vi "daqio_Fire_Event.vi"(7 "Event Key":string, 8 "error in (no error)":errorcluster, 9 "Event Value":string, 10 "Event Date and Time":timestamp, 11 "daq.io type in":T1={"daq.io ref"=refnum, "daq.io API Base"="http://dashboard.daq.io/api/v1", "Device Type Key"="", "Device Key"="", "Account ID"="", "online"=FALSE}) -> (0 "error out":errorcluster, 3 "daq.io type out":T1={"daq.io ref"=refnum, "daq.io API Base"="http://dashboard.daq.io/api/v1", "Device Type Key"="", "Device Key"="", "Account ID"="", "online"=FALSE})   [LabVIEW 2013, in "daqio minimal.lvlib"]
doc: "This VI will Fire an Event for the given Event Key. If the Event Key does not exist, it will create a new Event on the device. Every event fired will have a timestamp and a value associated with it. Events can be of any type and will be reflected on the \"Events\" page on daq.io. to retrieve all events that occured, use \"Get Device Events\"."
uses:
  daqio minimal.lvlib
  <vilib>/Easy HTTP Client/HTTP Header.ctl
  _typedefs/daqio-Type.ctl
  <vilib>/httpClient/ClientHandle.ctl
  _typedefs/daqio-Event-Def-Min.ctl
  _typedefs/FGV_commands.ctl
  _typedefs/daqio-Buffer-Commands.ctl
  <vilib>/Easy HTTP Client/Easy HTTP.lvlib
  <vilib>/httpClient/LabVIEWHTTPClient.lvlib
panel:
  out "JSON string":string
  out "headers":T3[](array[typedef])
  out "body":string
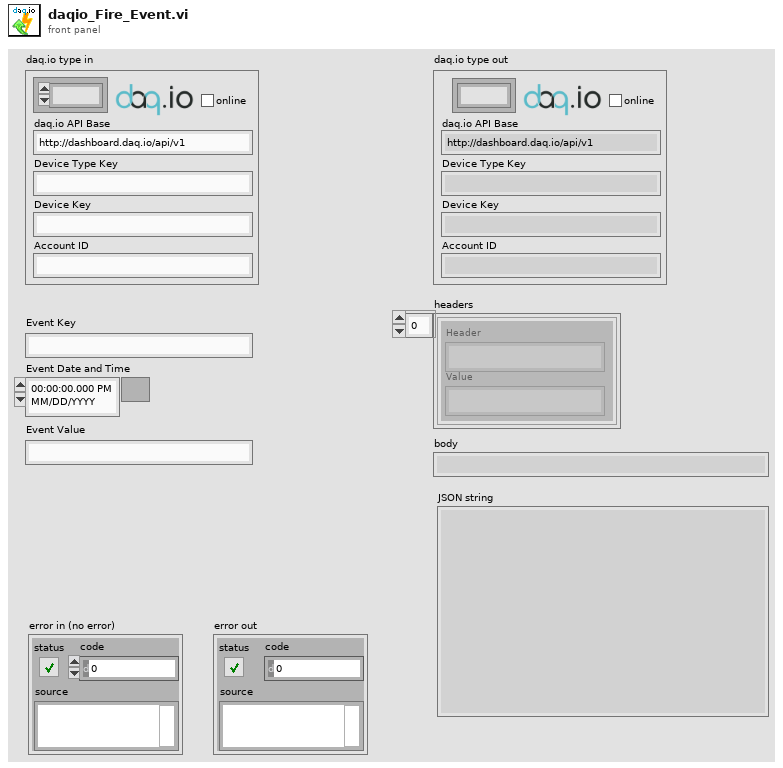
[diagram p1: front panel]
types:
  T1 = typedef "daqio minimal.lvlib/daqio-Type.ctl" = cluster{"daq.io ref":T2, "daq.io API Base":string, "Device Type Key":string, "Device Key":string, "Account ID":string, "online":bool}
  T2 = typedef "LabVIEWHTTPClient.lvlib/ClientHandle.ctl" = refnum<k1>
  T3 = typedef "Easy HTTP.lvlib/HTTP Header.ctl" = cluster{"Header":string, "Value":string}
  T4 = typedef "daqio minimal.lvlib/FGV_commands.ctl" = enum16{"Init / update", "Edit Item", "Find or Add Item", "Remove Item", "Delete All"}
  T5 = typedef "daqio minimal.lvlib/daqio-Event-Def-Min.ctl" = cluster{"event_type":string, "time":string, "value":string}
  T6 = typedef "daqio minimal.lvlib/daqio-Buffer-Commands.ctl" = enum16{"Add to Buffer", "Post from Buffer", "Clear Buffer", "Init"}
  T7 = typedef "daqio minimal.lvlib/daqio-Device-Type-Info-return.ctl" = cluster{"channel_types":T8[], "devices":T9[], "label":string, "event_types":T10[], "key":string, "tag_types":T11[], "id":string, "permissions":cluster{"write":string[], "read":string[]}}
  T8 = typedef "daqio minimal.lvlib/daqio-Channel-Type-POST-return.ctl" = cluster{"device_type_id":string, "id":string, "key":string, "label":string, "data_type":string, "permissions":cluster{"write":string[], "read":string[]}}
  T9 = typedef "daqio minimal.lvlib/daqio-Device.ctl" = cluster{"permissions":cluster{"write":string[], "read":string[]}, "id":string, "label":string, "key":string, "device_type_id":string, "tags":cluster{"key":string, "value":string}[], "files":string[]}
  T10 = typedef "daqio minimal.lvlib/daqio-Event-Type.ctl" = cluster{"device_type_id":string, "permissions":cluster{"read":string[], "write":string[]}, "id":string, "key":string, "label":string}
  T11 = typedef "daqio minimal.lvlib/daqio-Tag-Type-POST-return.ctl" = cluster{"label":string, "id":string, "device_type_id":string, "permissions":cluster{"write":string[], "read":string[]}, "default":string, "key":string}
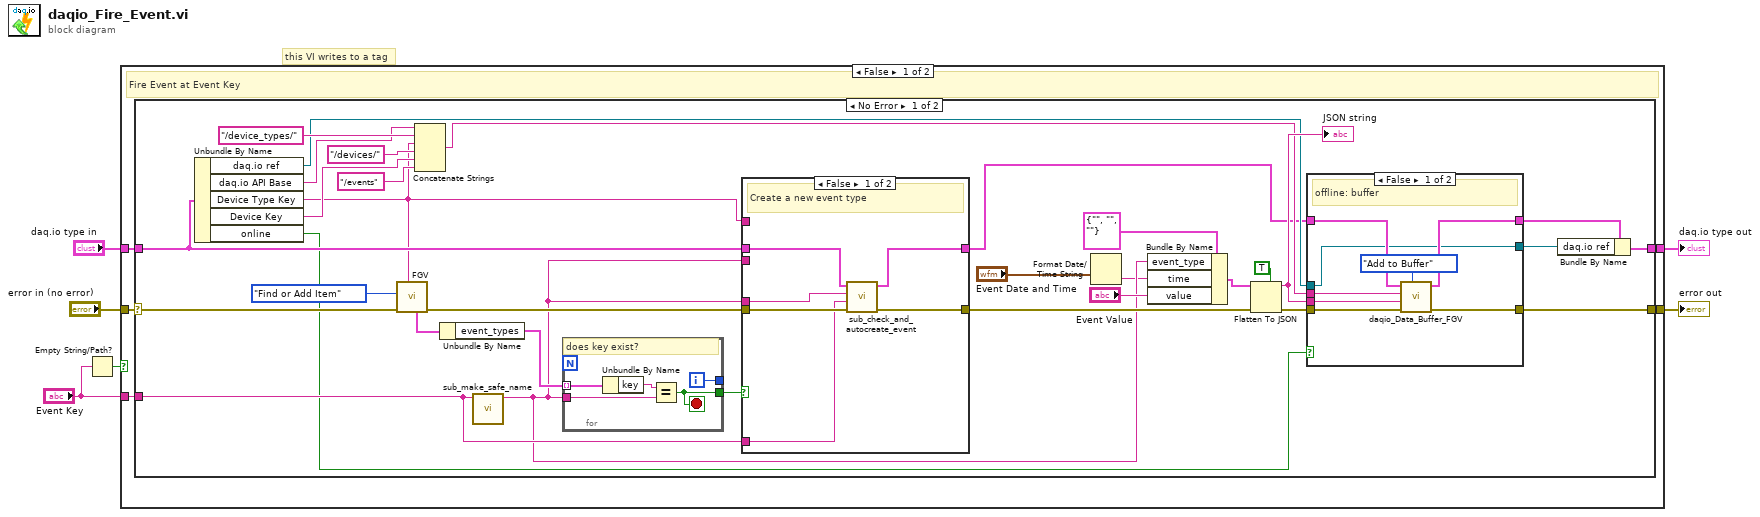
[diagram p0: block diagram]
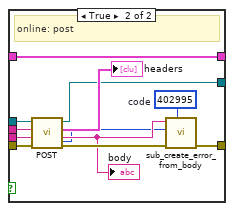
[diagram p2: hidden frame]
diagram:
  # "this VI writes to a tag"
  n1 = Empty String/Path?(string/path="Event Key") -> (empty?=w2:bool)
  n2 = case shown="False" w2 {
    tunnel: [w11 w80] -> w6
    tunnel: [w10 w79] -> w5
    tunnel: "error in (no error)" -> [w9 w79]
    tunnel: "daq.io type in" -> [w8 w80]
    tunnel: "Event Key" -> [w7 _]
    frame False {
      # "Fire Event at Event Key"
      n3 = case shown="No Error" w9 {
        selector: w9 -> [w27 w77]
        tunnel: [w35 w78] -> w11
        tunnel: [w33 w77] -> w10
        tunnel: w8 -> [w26 w78]
        tunnel: w7 -> [w18 _]
        frame No Error {
          n4 = Unbundle By Name(w26) -> ("daq.io ref"=w37:T2, "daq.io API Base"=w34:string, "Device Type Key"=w24:string, "Device Key"=w32:string, "online"=w16:bool)
          n5 = call "FGV.vi"("Dev Type Key"=w24, "error in (no error)"=w27, "Action"=FGV_commands."Find or Add Item") -> ("error out"=w28:errorcluster, "Dev Type out"=w29:T7)  [unwired: 4 in, 3 out]
          n6 = Concatenate Strings(w34, "/device_types/", w24, "/devices/", w32, "/events") -> (w41:string)
          n7 = Unbundle By Name(w29) -> ("event_types"=w23:T10[])
          n8 = call "sub_make_safe_name.vi"("Input String"=w18) -> ("Safe Output String"=w17:string)  [unwired: 10 in]
          n9 = for {
            tunnel: w23 -> [w76] mode=indexing
            tunnel: w17 -> [w74]
            tunnel: [w73] -> w25
            tunnel: [w72] -> _
            i -> [w72]
            stop <- w73 stop-if-true
            # "does key exist?"
            n10 = Unbundle By Name(w76) -> ("key"=w75:string)
            n11 = Equal?(x=w75, y=w74) -> (x = y?=w73:bool)
          }
          n12 = case shown="False" w25 {
            tunnel: w17 -> [w66 _]
            tunnel: w28 -> [w69 w71]
            tunnel: w26 -> [w68 w70]
            tunnel: [w67 w70] -> w15
            tunnel: [w64 w71] -> w20
            tunnel: w24 -> [_ _]
            tunnel: w17 -> [_ _]
            tunnel: w18 -> [w65 _]
            frame False {
              # "Create a new event type"
              n13 = call "sub_check_and_autocreate_event.vi"("error in (no error)"=w69, "new Event Label"=w65, "Event Key to Create or Update"=w66, "daq.io type in in"=w68) -> ("error out"=w64:errorcluster, "daq.io type out"=w67:T1)  [unwired: 5 in, 1 out]
            }
            frame True {
              # "Key was found in the existing device types"
            }
          }
          n14 = Format Date/Time String(seconds (now)="Event Date and Time") -> (date/time string=w13:string)  [unwired: 2 in]
          n15 = Bundle By Name(cluster=T5 {"event_type"="", "time"="", "value"=""} ("Devices"), "event_type"=w17, "time"=w13, "value"="Event Value") -> (w21:T5)
          n16 = Flatten To JSON(enable LabVIEW extensions? (T)=TRUE, anything=w21, error in (no error)=w20) -> (JSON string=w42:string, 11:w43:errorcluster)
          "JSON string" <- w42
          n17 = case shown="False" w16 {
            tunnel: w43 -> [w49 w63]
            tunnel: w42 -> [w46 w61]
            tunnel: w41 -> [w47 w60]
            tunnel: w37 -> [w44 w59]
            tunnel: [w44 w58] -> w36
            tunnel: [w48 w55] -> w33
            tunnel: w15 -> [w51 w52]
            tunnel: [w50 w52] -> w14
            frame False {
              # "offline: buffer"
              n18 = call "daqio_Data_Buffer_FGV.vi"("Buffer Command"=daqio-Buffer-Commands."Add to Buffer", "error in (no error)"=w49, "JSON Data"=w46, "API route"=w47, "daq.io type in"=w51) -> ("error out"=w48:errorcluster, "daq.io type out"=w50:T1)  [unwired: 5 in]
            }
            frame True {
              w54 = 402995  # code
              # "online: post"
              n19 = call <vilib>:"POST.vi"("error in (no error)"=w63, "data"=w61, "url"=w60, "client handle"=w59) -> ("error out"=w57:errorcluster, "body"=w56:string, "headers"=→"headers":T3[], "client handle out"=w58:T2, "HTTP Response Code"=w53:i32)  [unwired: 3 in]
              "body" <- w56
              n20 = call "sub_create_error_from_body.vi"("error code"=w54, "error in (no error)"=w57, "http code"=w53, "body"=w56) -> ("error out"=w55:errorcluster)  [unwired: 7 in]
            }
          }
          n21 = Bundle By Name(cluster=w14, "daq.io ref"=w36) -> (w35:T1)
        }
        frame Error {
        }
      }
    }
    frame True {
      # "No Event Key given, nothing to do"
    }
  }
  "error out" <- w5
  "daq.io type out" <- w6
